vi "Convert pData to TIFF.vi"(6 "Img Dst Array":T1[](array[typedef]), 7 "pDataBuffer":u16[](array[numeric]), 10 "Paths for TIFFs":path[](array[path]), 11 "Confocal Controls":T2 {"Field Size" min=5.0 max=255.0 step=1.0 scale=5.0..255.0; "Field Size in um" min=1.0 max=300.0 step=0.1; "MicronsPerPx" min=0.01 step=0.01 format="%.2f"; "Gain"."Gain B" min=1 max=100 step=1; "Gain"."Gain A" min=1 max=100 step=1; "Voltage Range"."Range B" items=["100mV"=5, "200mV"=6, "400mV"=7, "1V"=10, "2V"=11, "4V"=12]; "Voltage Range"."Range A" items=["100mV"=5, "200mV"=6, "400mV"=7, "1V"=10, "2V"=11, "4V"=12]; "Pixel Count"."Pixels in Y" items=["32"=32, "64"=64, "128"=128, "256"=256, "512"=512, "1024"=1024, "2048"=2048]; "Pixel Count"."Pixels in X" items=["32"=32, "64"=64, "128"=128, "256"=256, "512"=512, "1024"=1024, "2048"=2048]}) -> (4 "Img Dst Array out":T1[](array[typedef]))   [LabVIEW 2020]
uses:
  _Controls/Confocal Controls.ctl
  <vilib>/vision/Image Controls.llb/IMAQ Image.ctl
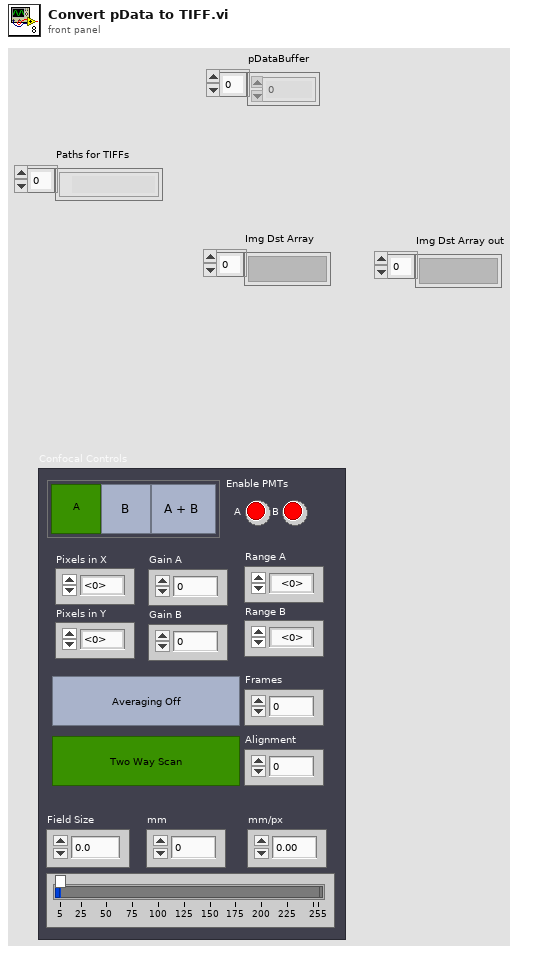
[diagram p1: front panel]
types:
  T1 = typedef "IMAQ Image.ctl" = refnum<image>
  T2 = typedef "Confocal Controls.ctl" = cluster{"Channel Selection":enum32{"A", "B", "AB"}, "Pixel Count":cluster{"Pixels in X":u32, "Pixels in Y":u32}, "Field Size":dbl, "Frames":u8, "Averaging":bool, "Alignment":dbl, "Scan Mode":bool, "Gain":cluster{"Gain A":u8, "Gain B":u8}, "Enable PMTs":cluster{"A":bool, "B":bool}, "Voltage Range":cluster{"Range A":u16, "Range B":u16}, "Multi Frame Count":dbl, "Trigger Mode":dbl, "Real Time Averaging":bool, "Field Size in um":dbl, "MicronsPerPx":dbl}
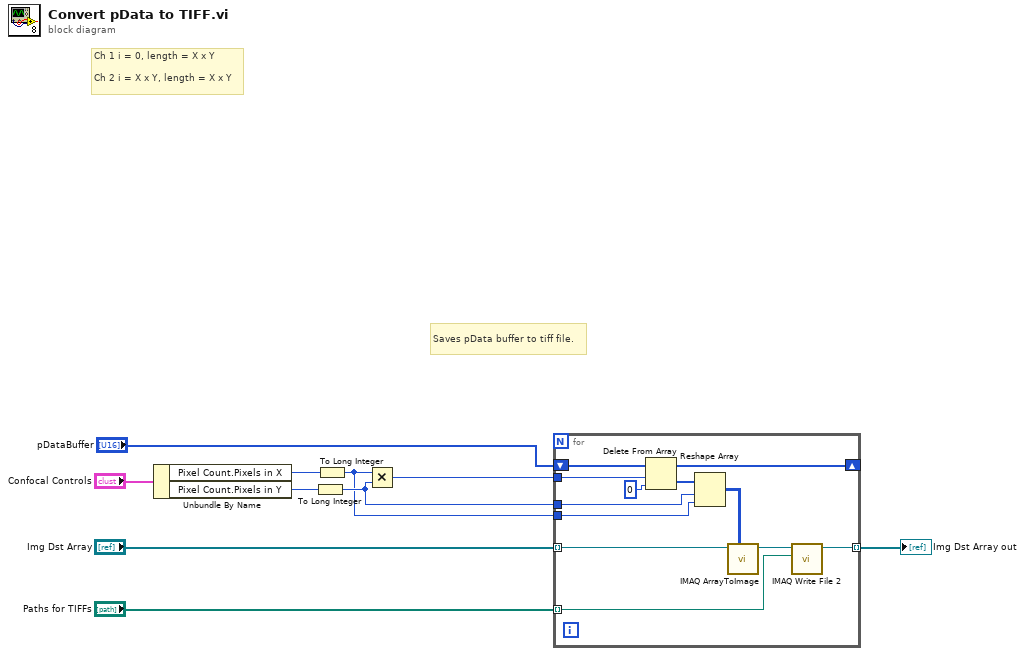
[diagram p0: block diagram]
diagram:
  # "Saves pData buffer to tiff file."
  # "Ch 1 i = 0, length = X x Y\n\nCh 2 i = X x Y, length = X x Y"
  n1 = Unbundle By Name("Confocal Controls") -> ("Pixel Count.Pixels in X"=w8:u32, "Pixel Count.Pixels in Y"=w9:u32)
  n2 = To Long Integer(number=w9) -> (32bit integer=w7:i32)
  n3 = To Long Integer(number=w8) -> (32bit integer=w6:i32)
  n4 = Multiply(x=w6, y=w7) -> (x*y=w2:i32)
  n5 = for {
    tunnel: w2 -> [w14]
    tunnel: w7 -> [w22]
    tunnel: w6 -> [w21]
    tunnel: "Img Dst Array" -> [w19] mode=indexing
    tunnel: [w17] -> w4 mode=indexing
    shift-right: [w12] -> _
    shift-left: "pDataBuffer" -> [w16]
    tunnel: "Paths for TIFFs" -> [w11] mode=indexing
    n6 = Delete From Array(array=w16, length=w14, index=0) -> (deleted portion=w13:u16[], array with subset deleted=w12:u16[])
    n7 = Reshape Array(w13, w22, w21) -> (w20:u16[][])
    n8 = call "IMAQ ArrayToImage"("Image Pixels (U16)"=w20, "Image"=w19) -> ("Image Out"=w18:T1)  [unwired: 8 in, 1 out]
    n9 = call-poly "IMAQ Write File 2"("File Path"=w11, "Image"=w18) -> ("Image Out (duplicate)"=w17:T1)  [unwired: 8 in, 1 out]
  }
  "Img Dst Array out" <- w4
